vi "解一元二次方程2（完成复数计算）.vi"() -> ()   [LabVIEW 2018]
panel:
  out "第二个解":cdb
  out "第一个解":cdb
  in  "D":dbl
  in  "C":dbl
  in  "B":dbl
  in  "A":dbl
  # "AX2+BX+C=D"
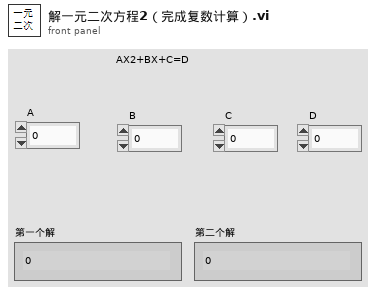
[diagram p1: front panel]
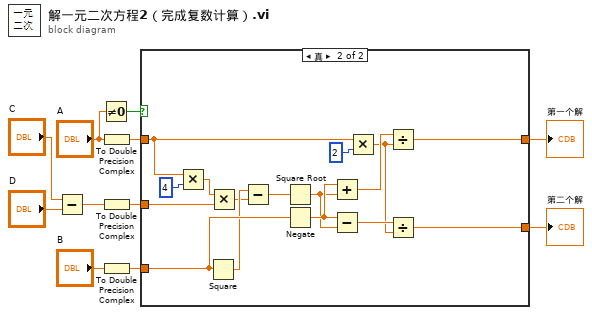
[diagram p0: block diagram]
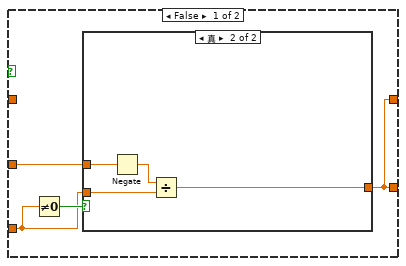
[diagram p2: hidden frame]
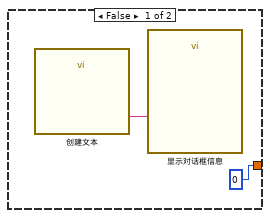
[diagram p3: hidden frame]
diagram:
  n1 = Subtract(x="C", y="D") -> (x-y=w4:dbl)
  n2 = Not Equal To 0?(x="A") -> (x != 0?=w5:bool)
  n3 = To Double Precision Complex(1:"A") -> (0:w9:cdb)
  n4 = To Double Precision Complex(1:w4) -> (0:w3:cdb)
  n5 = To Double Precision Complex(1:"B") -> (0:w7:cdb)
  n6 = case shown="真" w5 {
    tunnel: w9 -> [_ w26]
    tunnel: w7 -> [w13 w36]
    tunnel: w3 -> [w14 w32]
    tunnel: [w12 w23] -> w2
    tunnel: [w12 w22] -> w1
    frame False {
      n7 = Not Equal To 0?(x=w13) -> (x != 0?=w15:bool)
      n8 = case shown="真" w15 {
        tunnel: w14 -> [_ w21]
        tunnel: w13 -> [_ w19]
        tunnel: [0 w18] -> w12
        frame False {
          n9 = call "创建文本"() -> ("Result"=w16:string)  [unwired: 14 in, 1 out]
          n10 = call "显示对话框信息"("Message"=w16) -> ()  [unwired: 9 in, 2 out]
        }
        frame True {
          n11 = Negate(x=w21) -> (-x=w20:cdb)
          n12 = Divide(x=w20, y=w19) -> (x/y=w18:cdb)
        }
      }
    }
    frame True {
      n13 = Multiply(x=w26, y=4) -> (x*y=w33:cdb)
      n14 = Square(x=w36) -> (x^2=w35:cdb)
      n15 = Multiply(x=w33, y=w32) -> (x*y=w31:cdb)
      n16 = Subtract(x=w35, y=w31) -> (x-y=w30:cdb)
      n17 = Square Root(x=w30) -> (sqrt(x)=w29:cdb)
      n18 = Negate(x=w36) -> (-x=w37:cdb)
      n19 = Add(x=w37, y=w29) -> (x+y=w28:cdb)
      n20 = Subtract(x=w37, y=w29) -> (x-y=w27:cdb)
      n21 = Multiply(x=w26, y=2) -> (x*y=w24:cdb)
      n22 = Divide(x=w28, y=w24) -> (x/y=w23:cdb)
      n23 = Divide(x=w27, y=w24) -> (x/y=w22:cdb)
    }
  }
  "第一个解" <- w2
  "第二个解" <- w1
